vi "test variant to json path.vi"(8 "error in (no error)":errorcluster) -> (0 "error out":errorcluster)   [LabVIEW 2019, in "labview_json_tests.lvlib"]
uses:
  labview_json_tests.lvlib
  lib/labview_json.lvlib
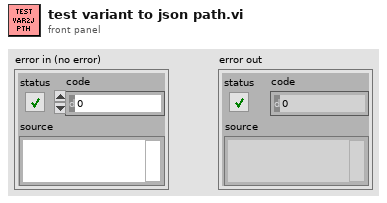
[diagram p1: front panel]
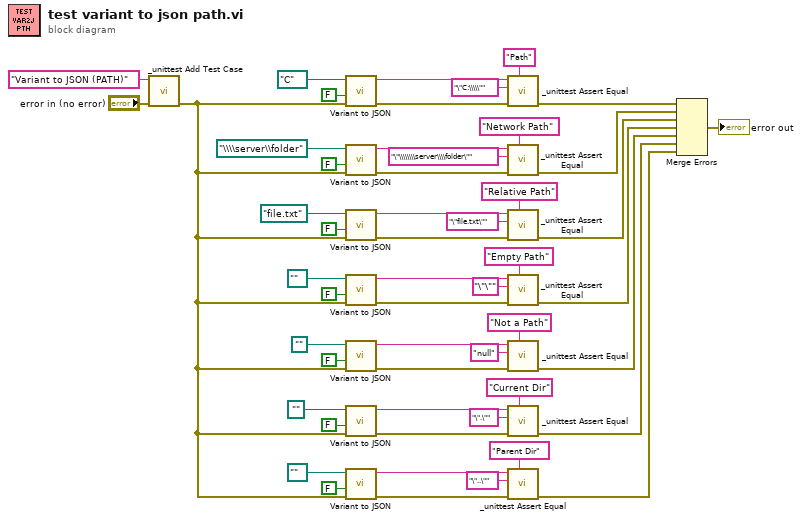
[diagram p0: block diagram]
diagram:
  n1 = call "_unittest Add Test Case.vi"("error in (no error)"="error in (no error)", "Test Case"="Variant to JSON (PATH)") -> ("error out"=w8:errorcluster)  [unwired: 9 in]
  n2 = call "Variant to JSON.vi"("error in (no error)"=w8, "Pretty Print? (F)"=FALSE, "Variant in"=path "C:/") -> ("error out"=w49:errorcluster, "JSON"=w48:string)  [unwired: 7 in]
  n3 = call "Variant to JSON.vi"("error in (no error)"=w8, "Pretty Print? (F)"=FALSE, "Variant in"=path "\\\\server\\folder") -> ("error out"=w41:errorcluster, "JSON"=w42:string)  [unwired: 7 in]
  n4 = call "Variant to JSON.vi"("error in (no error)"=w8, "Pretty Print? (F)"=FALSE, "Variant in"=path "file.txt") -> ("error out"=w37:errorcluster, "JSON"=w36:string)  [unwired: 7 in]
  n5 = call "Variant to JSON.vi"("error in (no error)"=w8, "Pretty Print? (F)"=FALSE, "Variant in"=path "") -> ("error out"=w29:errorcluster, "JSON"=w30:string)  [unwired: 7 in]
  n6 = call "Variant to JSON.vi"("error in (no error)"=w8, "Pretty Print? (F)"=FALSE, "Variant in"=path "" ("Not A Path Constant")) -> ("error out"=w25:errorcluster, "JSON"=w24:string)  [unwired: 7 in]
  n7 = call "Variant to JSON.vi"("error in (no error)"=w8, "Pretty Print? (F)"=FALSE, "Variant in"=path "") -> ("error out"=w19:errorcluster, "JSON"=w18:string)  [unwired: 7 in]
  n8 = call "Variant to JSON.vi"("error in (no error)"=w8, "Pretty Print? (F)"=FALSE, "Variant in"=path "..") -> ("error out"=w12:errorcluster, "JSON"=w13:string)  [unwired: 7 in]
  n9 = call "_unittest Assert Equal.vi"("Message"="Path", "error in (no error)"=w49, "Expected Value"="\"C:\\\\\"", "Actual Value"=w48) -> ("error out"=w46:errorcluster)  [unwired: 7 in]
  n10 = call "_unittest Assert Equal.vi"("Message"="Network Path", "error in (no error)"=w41, "Expected Value"="\"\\\\\\\\server\\\\folder\"", "Actual Value"=w42) -> ("error out"=w39:errorcluster)  [unwired: 7 in]
  n11 = call "_unittest Assert Equal.vi"("Message"="Relative Path", "error in (no error)"=w37, "Expected Value"="\"file.txt\"", "Actual Value"=w36) -> ("error out"=w33:errorcluster)  [unwired: 7 in]
  n12 = call "_unittest Assert Equal.vi"("Message"="Empty Path", "error in (no error)"=w29, "Expected Value"="\"\"", "Actual Value"=w30) -> ("error out"=w27:errorcluster)  [unwired: 7 in]
  n13 = call "_unittest Assert Equal.vi"("Message"="Not a Path", "error in (no error)"=w25, "Expected Value"="null", "Actual Value"=w24) -> ("error out"=w22:errorcluster)  [unwired: 7 in]
  n14 = call "_unittest Assert Equal.vi"("Message"="Current Dir", "error in (no error)"=w19, "Expected Value"="\".\"", "Actual Value"=w18) -> ("error out"=w10:errorcluster)  [unwired: 7 in]
  n15 = call "_unittest Assert Equal.vi"("Message"="Parent Dir", "error in (no error)"=w12, "Expected Value"="\"..\"", "Actual Value"=w13) -> ("error out"=w9:errorcluster)  [unwired: 7 in]
  n16 = Merge Errors(w46, w39, w33, w27, w22, w10, w9) -> (→"error out":errorcluster)
